vi "GetEvents_GIS Printer.vi"(8 "error in (no error)":errorcluster, 11 "TopLevel in":refnum<class "GIS Printer.lvclass">) -> (0 "error out":errorcluster, 2 "UserEvents":T1, 3 "TopLevel out":refnum<class "GIS Printer.lvclass">)   [LabVIEW 2022 SP3, in "GIS Printer.lvclass"]
uses:
  GIS Printer.lvclass
  Typedefs/UserEvents.ctl
  Typedefs/API Event Data.ctl
  Typedefs/API Task State.ctl
  Typedefs/Status Cluster.ctl
  Typedefs/AbortEventData--Cluster.ctl
  Typedefs/GIS Status--Cluster.ctl
  Typedefs/HeadEnableStatus--cluster.ctl
  GIS Printer.lvclass/GIS Printer.ctl
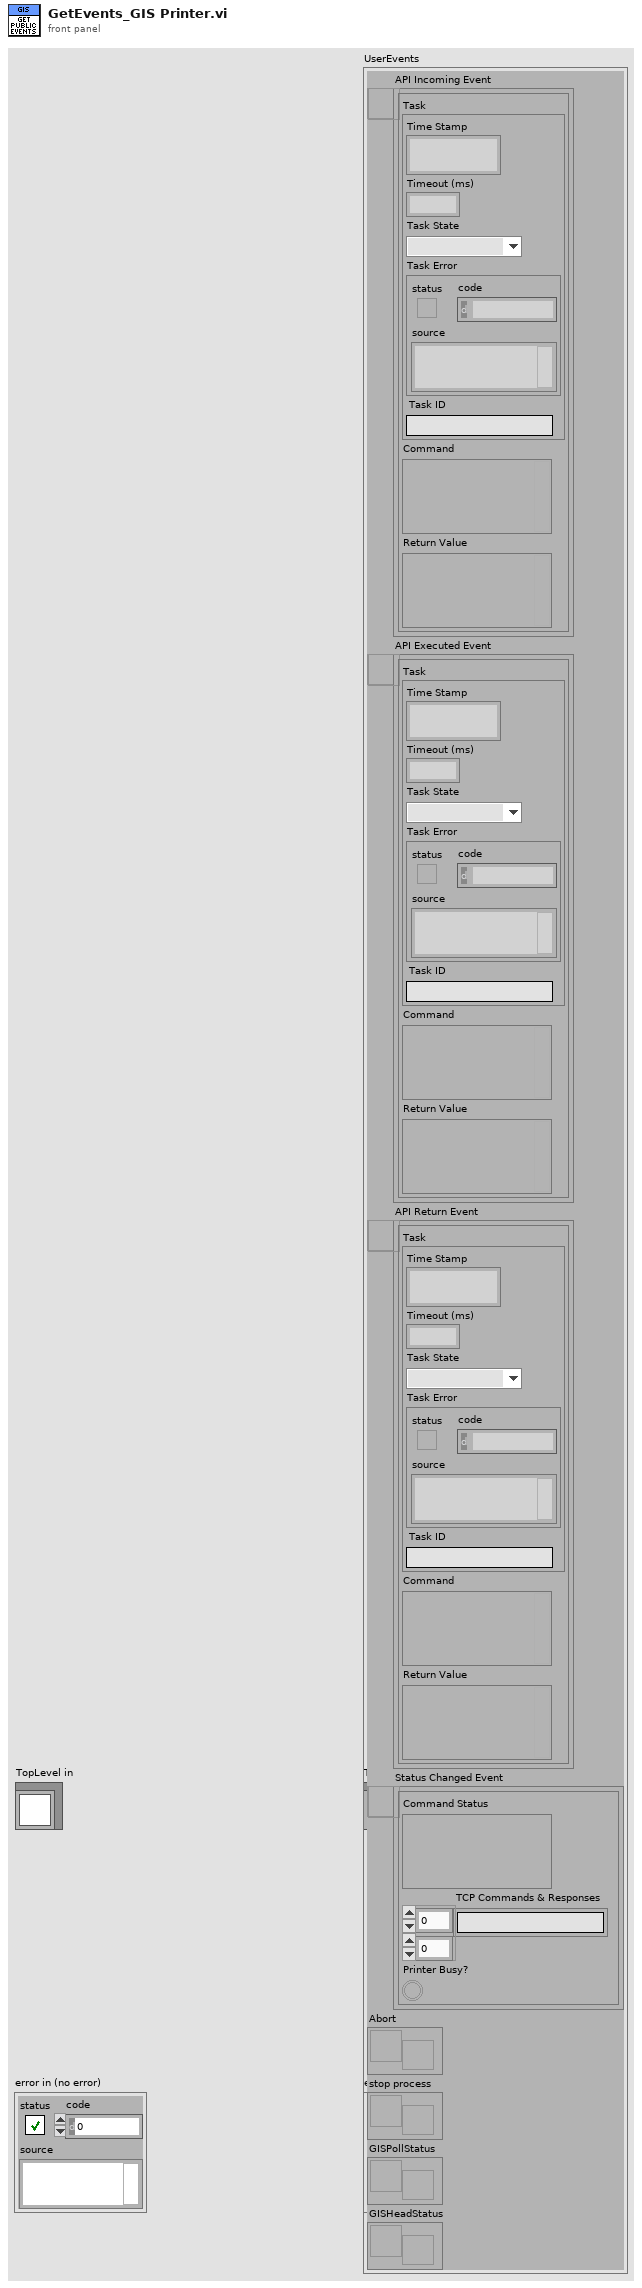
[diagram p1: front panel]
types:
  T1 = typedef "GIS Printer.lvclass/UserEvents.ctl" = cluster{"API Incoming Event":refnum<user-event>, "API Executed Event":refnum<user-event>, "API Return Event":refnum<user-event>, "Status Changed Event":refnum<user-event>, "Abort":refnum<user-event>, "stop process":refnum<user-event>, "GISPollStatus":refnum<user-event>, "GISHeadStatus":refnum<user-event>}
  T2 = typedef "GIS Printer.lvclass/Private Data.ctl" = cluster{"UserEvents":T1, "All Dependencies":cluster{"Class References":refnum<class>[], "Class Names":string[]}, "PrinterConiguration":T3, "Status":T4, "GISHeadStatus":T5[], "HeadStatus":T6}
  T3 = typedef "GIS Printer.lvclass/PrinterConfiguration--Cluster.ctl" = cluster{"IPAddress":string, "Move Stage on RTP Command?":bool, "Stage Move Position":string, "PH1-Prime Path":path, "PH2-Prime Path":path, "PH3-Prime Path":path, "PH4-Prime Path":path, "PH5-Prime Path":path, "PH6-Prime Path":path, "PrintScriptsFolder":path, "PurgeScriptsFolder":path, "StageScriptsFolder":path, "PH1-HeatOn Path":path, "PH2-HeatOn Path":path, "PH3-HeatOn Path":path, "PH4-HeatOn Path":path, "PH5-HeatOn Path":path, "PH6-HeatOn Path":path, "PH1-HeatOff Path":path, "PH2-HeatOff Path":path, "PH3-HeatOff Path":path, "PH4-HeatOff Path":path, "PH5-HeatOff Path":path, "PH6-HeatOff Path":path}
  T4 = typedef "GIS Printer.lvclass/Status Cluster.ctl" = cluster{"Command Status":variant, "TCP Commands & Responses":string[][], "Printer Busy?":bool}
  T5 = typedef "GIS Status--Cluster.ctl" = cluster{"HeadEnabled":bool, "SpitEnabled":bool, "HeaterEnabled":bool, "TargetTemperature":dbl, "CurrentTemperature":dbl}
  T6 = typedef "HeadEnableStatus--cluster.ctl" = cluster{"PH1_Enable":bool, "PH2_Enable":bool, "PH3_Enable":bool, "PH4_Enable":bool, "PH5_Enable":bool, "PH6_Enable":bool}
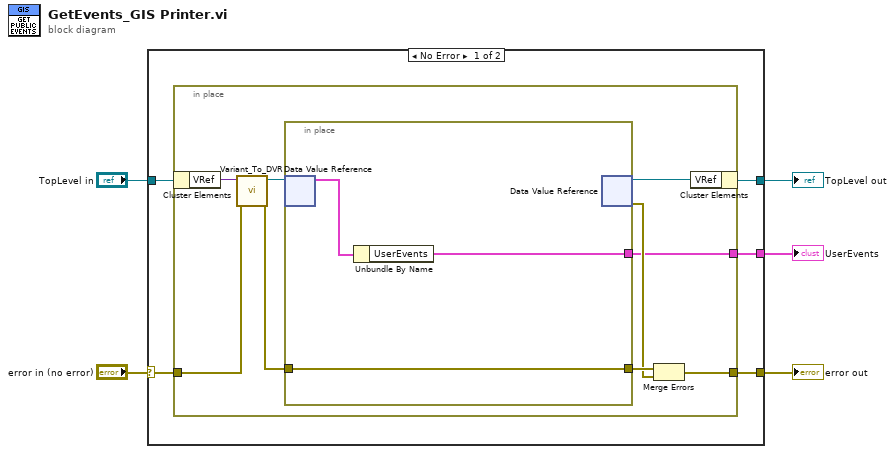
[diagram p0: block diagram]
diagram:
  n1 = case shown="No Error" "error in (no error)" {
    selector: "error in (no error)" -> [w7 w24]
    tunnel: [w9 w24] -> w4
    tunnel: [w10 w23] -> w2
    tunnel: "TopLevel in" -> [w8 w23]
    tunnel: [w6 _] -> w1
    frame No Error {
      n2 = in-place {
        in-place-border: w7 -> [w17]
        in-place-border: [w13] -> w9
        in-place-border: [w11] -> w6
        n3 = in-place-cluster #1(w8) -> ("VRef"=w19:variant)
        n4 = call "Variant_To_DVR.vi"("error in (no error)"=w17, "Variant"=w19) -> ("error out"=w16:errorcluster, "DVR"=w18:refnum<data-value>)  [unwired: 8 in]
        n5 = in-place {
          in-place-border: w16 -> [w21]
          in-place-border: [w21] -> w15
          in-place-border: [w20] -> w11
          n6 = in-place-dvr #2(w18) -> (w22:T2)  [unwired: 1 out]
          n7 = Unbundle By Name(w22) -> ("UserEvents"=w20:T1)
          n8 = in-place-dvr #2() -> (w12:refnum<data-value>, w14:errorcluster)  [unwired: 1 in]
        }
        n9 = Merge Errors(w15, w14) -> (w13:errorcluster)
        n10 = in-place-cluster #1("VRef"=w12) -> (w10:refnum<class "GIS Printer.lvclass">)
      }
    }
    frame Error {
    }
  }
  "error out" <- w4
  "TopLevel out" <- w2
  "UserEvents" <- w1
